vi "Change Camera.vi"(8 "error in (no error)":errorcluster, 10 "New Camera":string, 11 "HIJ Vision Camera App in":refnum<class "HIJ Vision Camera App.lvclass">) -> (0 "error out":errorcluster, 3 "HIJ Vision Camera App out":refnum<class "HIJ Vision Camera App.lvclass">)   [LabVIEW 2014, in "HIJ Vision Camera App.lvlib" / "HIJ Vision Camera App.lvclass"]
uses:
  HIJ Vision Camera App.lvclass
  HIJ Vision Camera App.lvclass/HIJ Vision Camera App.ctl
  HIJ Vision Application/HIJ Vision Application/HIJ Vision Application.lvclass/HIJ Vision Application.ctl
  Camera Actor/Camera Actor Messages/Change Camera Msg/Change Camera Msg.lvclass/Change Camera Msg.ctl
  <vilib>/ActorFramework/Message Enqueuer/Message Enqueuer.lvclass/Message Enqueuer.ctl
  HIJ Vision Display/HIJ Vision Display Messages/Change Image Source Msg/Change Image Source Msg.lvclass/Change Image Source Msg.ctl
  HIJ Vision Application/HIJ Vision Application/Read Display Enq.vi
  <vilib>/ActorFramework/Message Enqueuer/Enqueue.vi
  <vilib>/ActorFramework/Message Priority Queue/Priority Enqueue.vi
  <vilib>/ActorFramework/Message Enqueuer/Message Enqueuer.lvclass
  Camera Actor/Camera Actor Messages/Change Camera Msg/Change Camera Msg.lvclass
  HIJ Vision Display/HIJ Vision Display Messages/Change Image Source Msg/Change Image Source Msg.lvclass
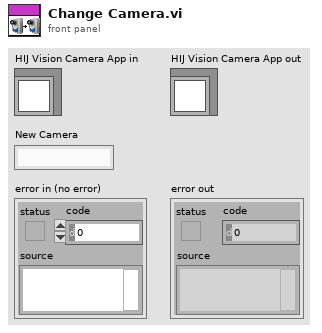
[diagram p1: front panel]
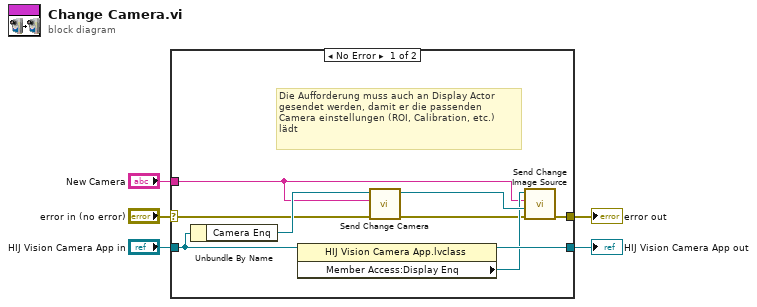
[diagram p0: block diagram]
diagram:
  n1 = case shown="No Error" "error in (no error)" {
    selector: "error in (no error)" -> [w8 w16]
    tunnel: [w7 w16] -> w4
    tunnel: [w13 w15] -> w2
    tunnel: "HIJ Vision Camera App in" -> [w12 w15]
    tunnel: "New Camera" -> [w6 _]
    frame No Error {
      # "Die Aufforderung muss auch an Display Actor\ngesendet werden, damit er die passenden \nCamera einstellungen (ROI, Calibration, etc.)\nlädt"
      n2 = Unbundle By Name(w12) -> ("Camera Enq"=w11:refnum<class "Message Enqueuer.lvclass">)
      n3 = property class="HIJ Vision Camera App.lvclass"(reference=w12) -> (reference out=w13:refnum<class "HIJ Vision Camera App.lvclass">, "Member Access:Display Enq"=w10:refnum<class "Message Enqueuer.lvclass">)  [unwired: 1 in, 1 out]
      n4 = call "Send Change Camera.vi"("error in (no error)"=w8, "New Camera"=w6, "Message Enqueuer"=w11) -> ("error out"=w9:errorcluster, "Message Enqueuer out"=w14:refnum<class "Message Enqueuer.lvclass">)  [unwired: 7 in]
      n5 = call "Send Change Image Source.vi"("error in (no error)"=w9, "Image Source Enq"=w14, "Image Source"=w6, "Message Enqueuer"=w10) -> ("error out"=w7:errorcluster)  [unwired: 6 in, 1 out]
    }
    frame Error {
    }
  }
  "error out" <- w4
  "HIJ Vision Camera App out" <- w2
